vi "Find Enemy.vi"(10 "View":i32[](array[numeric]), 11 "Team Index":i32) -> (2 "Direction":T1, 3 "Found Enemy?":bool, 5 "Enemy":i32)   [LabVIEW 2020, in "Common.lvlib"]
doc: "Reports whether an enemy is in the vicinity and some information about that enemy."
uses:
  Common.lvlib
  Type Defs/Direction Enum.ctl
  Type Defs/SB Type Defs.lvlib
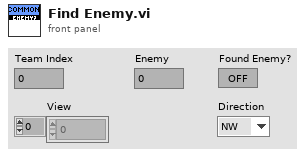
[diagram p1: front panel]
types:
  T1 = typedef "SB Type Defs.lvlib/Direction Enum.ctl" = enum16{"NW", "N", "NE", "E", "SE", "S", "SW", "W"}
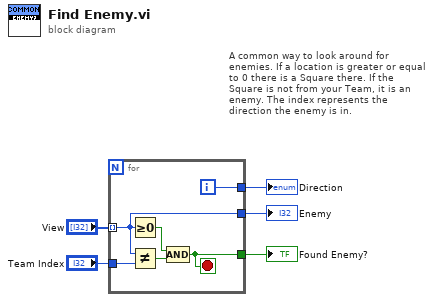
[diagram p0: block diagram]
diagram:
  # "A common way to look around for enemies. If a location is greater or equal to 0 there is a Square there. If the Square is not from your Team, it is an enemy. The index represents the direction the enemy is in."
  n1 = for {
    tunnel: "View" -> [w6] mode=indexing
    tunnel: "Team Index" -> [w10]
    tunnel: [w8] -> w5
    tunnel: [w7] -> w4
    tunnel: [w6] -> w1
    i -> [w8]
    stop <- w7 stop-if-true
    n2 = Greater Or Equal To 0?(x=w6) -> (x >= 0?=w11:bool)
    n3 = Not Equal?(x=w6, y=w10) -> (x != y?=w9:bool)
    n4 = Compound Arithmetic op=AND(w11, w9) -> (w7:bool)
  }
  "Direction" <- w5
  "Found Enemy?" <- w4
  "Enemy" <- w1
